vi "Project Step Operation.vi"(8 "error in (no error)":errorcluster, 9 "Drop Event Data":T1, 11 "Editor.lvclass in":refnum<data-value>) -> (0 "error out":errorcluster, 3 "Editor.lvclass out":refnum<data-value>)   [LabVIEW 2015, in "Editor.lvclass"]
uses:
  Editor.lvclass
  CallVIStep.lvclass
  CallEXEStep.lvclass
  UIStep.lvclass
  Project.lvclass
  Step.lvclass
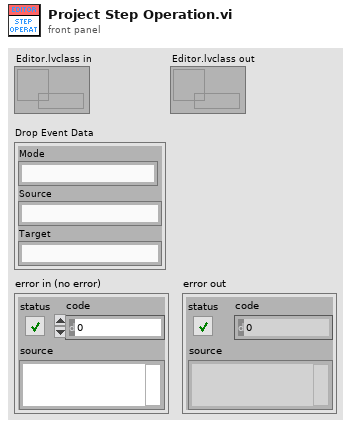
[diagram p1: front panel]
types:
  T1 = cluster{"Mode":string, "Source":string, "Target":string}
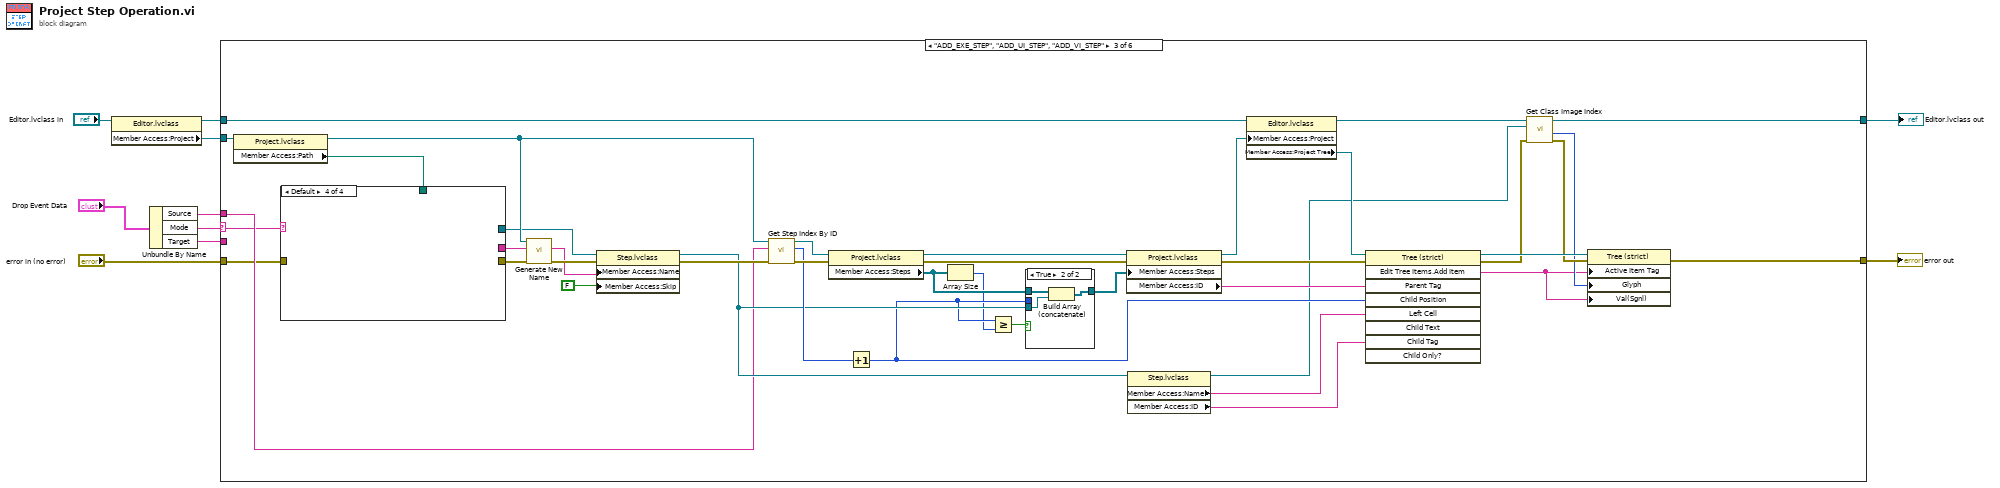
[diagram p0: block diagram]
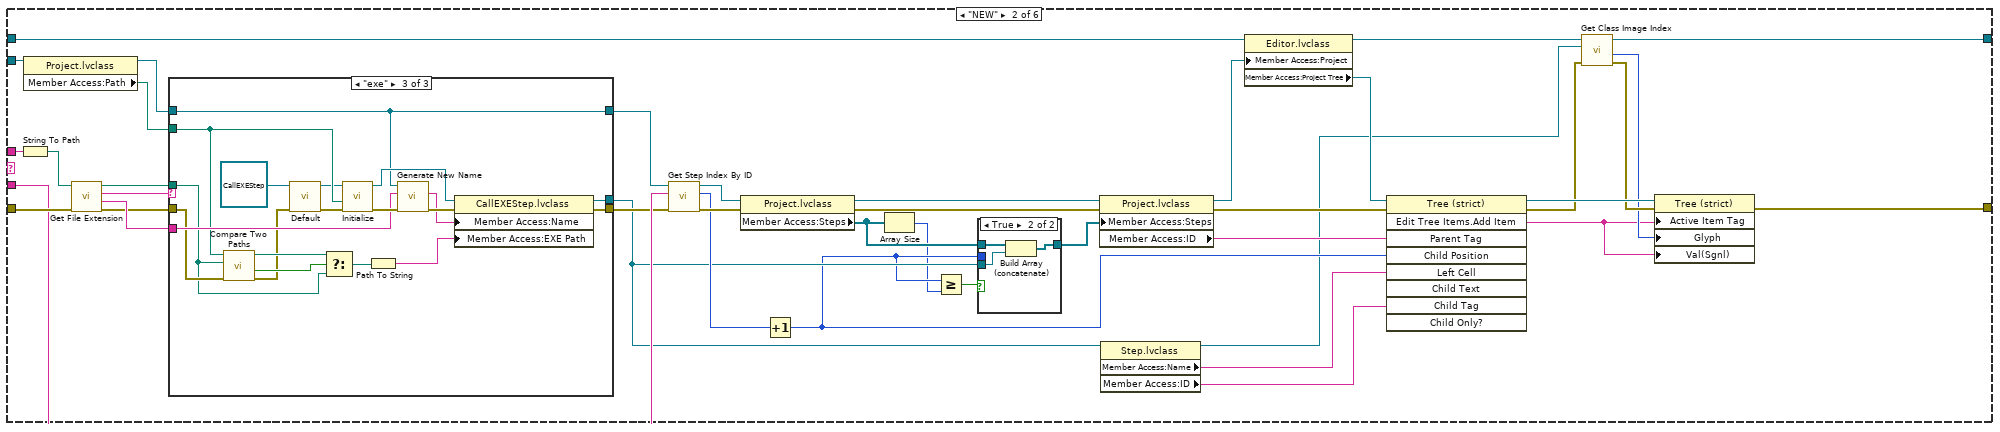
[diagram p3: hidden frame]
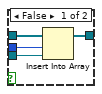
[diagram p4: hidden frame]
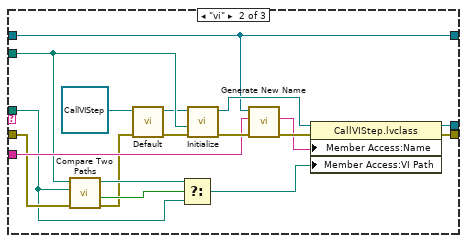
[diagram p6: hidden frame]
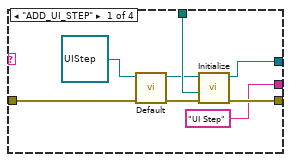
[diagram p7: hidden frame]
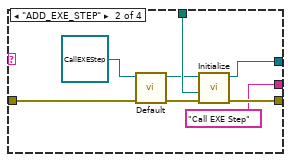
[diagram p8: hidden frame]
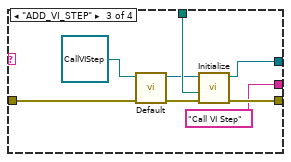
[diagram p9: hidden frame]
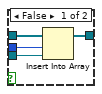
[diagram p10: hidden frame]
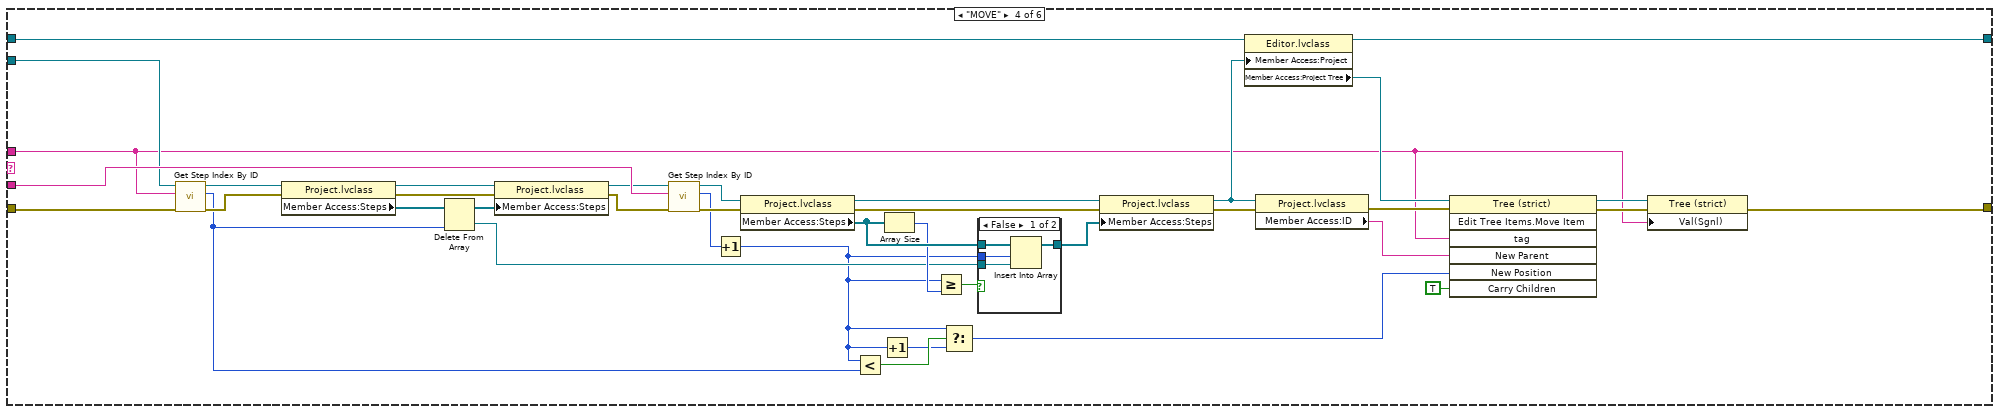
[diagram p11: hidden frame]
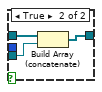
[diagram p12: hidden frame]
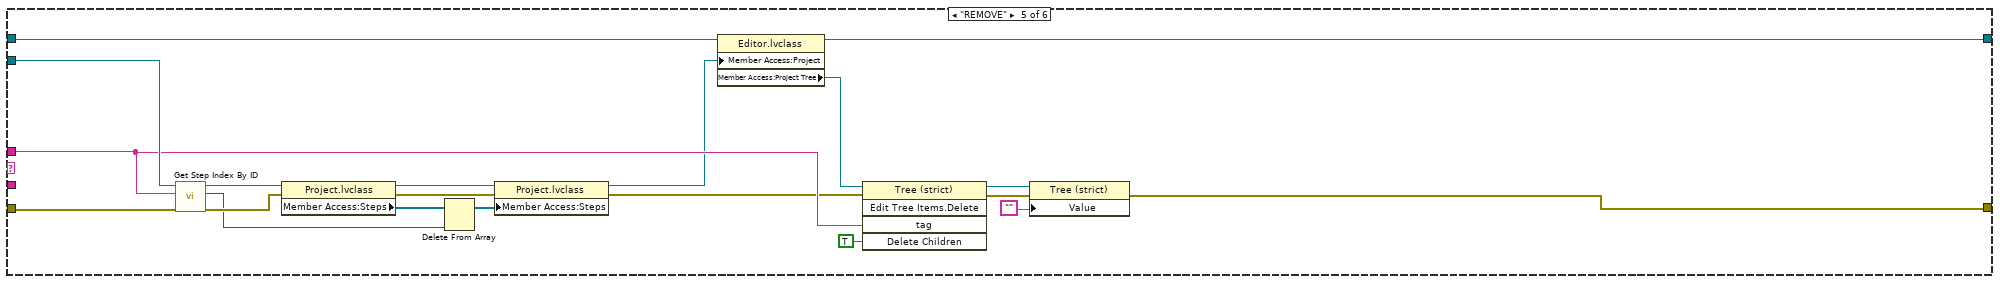
[diagram p13: hidden frame]
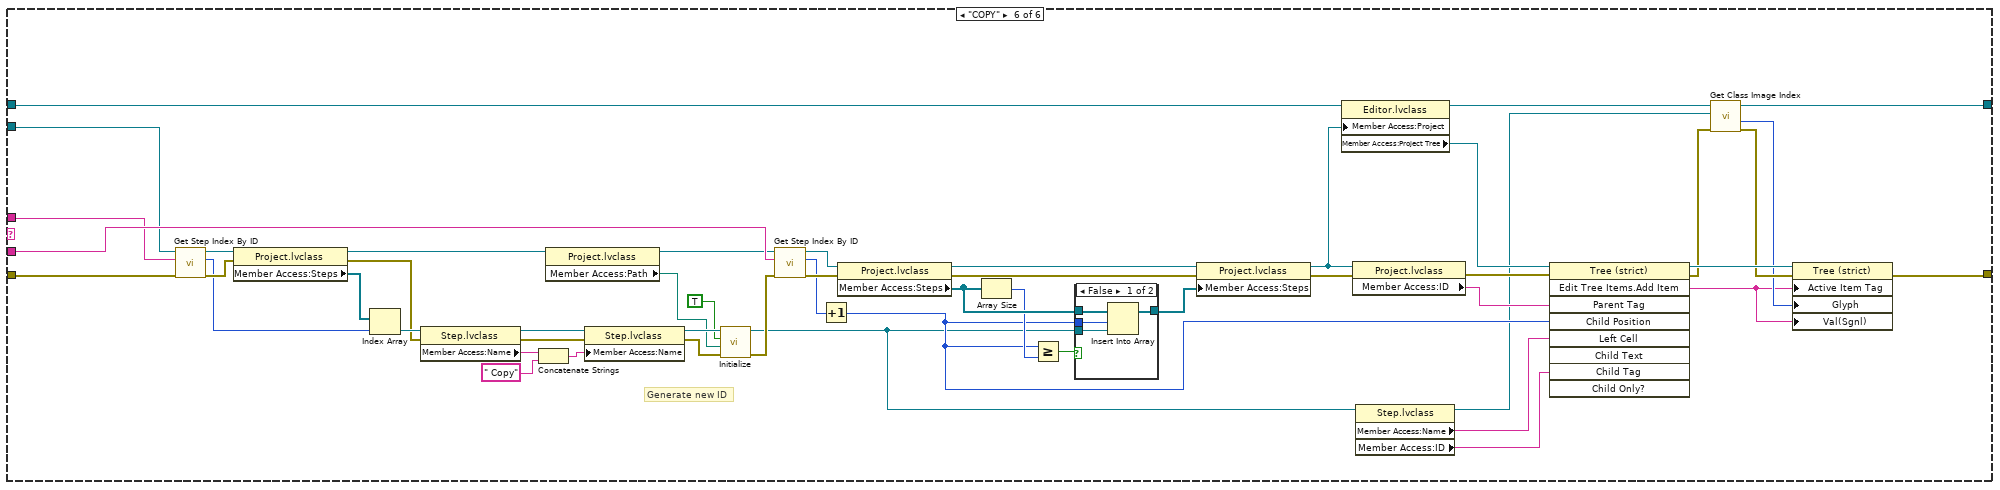
[diagram p14: hidden frame]
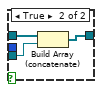
[diagram p15: hidden frame]
diagram:
  n1 = property class="Editor.lvclass"(reference="Editor.lvclass in") -> (reference out=w3:refnum<data-value>, "Member Access:Project"=w4:refnum<class "Project.lvclass">)  [unwired: 1 in, 1 out]
  n2 = Unbundle By Name("Drop Event Data") -> ("Source"=w8:string, "Mode"=w9:string, "Target"=w6:string)
  n3 = case shown="\"ADD_EXE_STEP\", \"ADD_UI_STEP\", \"ADD_VI_STEP\"" w9 {
    selector: w9 -> [_ _ w99 _ _ _]
    tunnel: w8 -> [_ w47 w102 w170 w219 w262]
    tunnel: w4 -> [_ w15 w109 w195 w232 w272]
    tunnel: "error in (no error)" -> [w11 w46 w100 w191 w228 w268]
    tunnel: w6 -> [_ w37 _ w200 _ w277]
    tunnel: w3 -> [w12 w45 w138 w207 w234 w284]
    tunnel: [w12 w17 w111 w184 w224 w242] -> w2
    tunnel: [w11 w16 w110 w171 w220 w263] -> w1
    frame Default {
    }
    frame "NEW" {
      n4 = String To Path(string=w47) -> (path=w48:path)
      n5 = property class="Project.lvclass"(reference=w15) -> (reference out=w14:refnum<class "Project.lvclass">, "Member Access:Path"=w13:path)  [unwired: 1 in, 1 out]
      n6 = call <vilib>:"Get File Extension.vi"("error in (no error)"=w46, "file"=w48) -> ("error out"=w50:errorcluster, "filename without extension"=w52:string, "lowercase file extension"=w49:string, "dup file"=w51:path)  [unwired: 5 in, 1 out]
      n7 = case shown="\"exe\"" w49 {
        tunnel: w50 -> [w61 w72 w91]
        tunnel: w51 -> [_ w67 w86]
        tunnel: [w61 w73 w92] -> w36
        tunnel: w14 -> [w60 w71 w90]
        tunnel: [w60 w71 w90] -> w38
        tunnel: w52 -> [_ w75 w94]
        tunnel: [_ w74 w93] -> w31
        tunnel: w13 -> [_ w70 w89]
        frame Default {
        }
        frame "vi" {
          n8 = call <vilib>:"Compare Two Paths.vi"("error in (no error)"=w72, "Path 2"=w67, "Path 1"=w70) -> ("error out"=w63:errorcluster, "Path 2 Relative to Path 1?"=w69:bool, "Relative Path from 1 to 2"=w68:path)  [unwired: 5 in, 1 out]
          n9 = call-dynamic "Default.vi"("error in (no error)"=w63, "CallVIStep in"=refnum<class "CallVIStep.lvclass"> refnum ("CallVIStep.lvclass")) -> ("error out"=w62:errorcluster, "CallVIStep out"=w64:refnum<class "CallVIStep.lvclass">)  [unwired: 8 in]
          n10 = Select(t=w68, s=w69, f=w67) -> (s? t:f=w66:path)
          n11 = call-dynamic "Initialize.vi"("error in (no error)"=w62, "Project Path"=w70, "Step in"=w64) -> ("error out"=w78:errorcluster, "Step out"=w79:refnum<class "CallVIStep.lvclass">)  [unwired: 7 in]
          n12 = call "Generate New Name.vi"("error in (no error)"=w78, "Default Name"=w75, "Project in"=w71) -> ("error out"=w77:errorcluster, "Name"=w76:string)  [unwired: 6 in, 1 out]
          n13 = property class="CallVIStep.lvclass"(reference=w79, error in=w77, "Member Access:Name"=w76, "Member Access:VI Path"=w66) -> (reference out=w74:refnum<class "CallVIStep.lvclass">, error out=w73:errorcluster)
        }
        frame "exe" {
          n14 = call <vilib>:"Compare Two Paths.vi"("error in (no error)"=w91, "Path 2"=w86, "Path 1"=w89) -> ("error out"=w81:errorcluster, "Path 2 Relative to Path 1?"=w87:bool, "Relative Path from 1 to 2"=w88:path)  [unwired: 5 in, 1 out]
          n15 = call-dynamic "Default.vi"("error in (no error)"=w81, "CallEXEStep in"=refnum<class "CallEXEStep.lvclass"> refnum ("CallEXEStep.lvclass")) -> ("error out"=w80:errorcluster, "CallEXEStep out"=w82:refnum<class "CallEXEStep.lvclass">)  [unwired: 8 in]
          n16 = Select(t=w88, s=w87, f=w86) -> (s? t:f=w85:path)
          n17 = call-dynamic "Initialize.vi"("error in (no error)"=w80, "Project Path"=w89, "Step in"=w82) -> ("error out"=w97:errorcluster, "Step out"=w98:refnum<class "CallEXEStep.lvclass">)  [unwired: 7 in]
          n18 = Path To String(path=w85) -> (string=w84:string)
          n19 = call "Generate New Name.vi"("error in (no error)"=w97, "Default Name"=w94, "Project in"=w90) -> ("error out"=w96:errorcluster, "Name"=w95:string)  [unwired: 6 in, 1 out]
          n20 = property class="CallEXEStep.lvclass"(reference=w98, error in=w96, "Member Access:Name"=w95, "Member Access:EXE Path"=w84) -> (reference out=w93:refnum<class "CallEXEStep.lvclass">, error out=w92:errorcluster)
        }
      }
      n21 = call "Get Step Index By ID.vi"("error in (no error)"=w36, "ID"=w37, "Project in"=w38) -> ("error out"=w41:errorcluster, "Index"=w40:i32, "Project out"=w42:refnum<class "Project.lvclass">)  [unwired: 6 in]
      n22 = property class="Project.lvclass"(reference=w42, error in=w41) -> (reference out=w44:refnum<class "Project.lvclass">, error out=w43:errorcluster, "Member Access:Steps"=w23:refnum<class "Step.lvclass">[])
      n23 = Increment(x=w40) -> (x+1=w21:i32)
      n24 = Array Size(array=w23) -> (size(s)=w20:i32)
      n25 = Greater Or Equal?(x=w21, y=w20) -> (x >= y?=w22:bool)
      n26 = case shown="True" w22 {
        tunnel: [w56 w57] -> w39
        tunnel: w31 -> [w55 w58]
        tunnel: w21 -> [w54 _]
        tunnel: w23 -> [w53 w59]
        frame False {
          n27 = Insert Into Array(array=w53, index=w54, new element=w55) -> (w56:refnum<class "Step.lvclass">[])
        }
        frame True {
          n28 = Build Array (concatenate)(w59, w58) -> (w57:refnum<class "Step.lvclass">[])
        }
      }
      n29 = property class="Project.lvclass"(reference=w44, error in=w43, "Member Access:Steps"=w39) -> (reference out=w35:refnum<class "Project.lvclass">, error out=w33:errorcluster, "Member Access:ID"=w32:string)
      n30 = property class="Step.lvclass"(reference=w31) -> (reference out=w18:refnum<class "Step.lvclass">, "Member Access:Name"=w30:string, "Member Access:ID"=w29:string)  [unwired: 1 in, 1 out]
      n31 = property class="Editor.lvclass"(reference=w45, "Member Access:Project"=w35) -> (reference out=w27:refnum<data-value>, "Member Access:Project Tree"=w34:refnum<vi>)  [unwired: 1 in, 1 out]
      n32 = invoke class="Tree (strict)" method="Edit Tree Items.Add Item"(reference=w34, error in=w33, "Parent Tag"=w32, "Child Position"=w21, "Left Cell"=w30, "Child Tag"=w29) -> (reference out=w28:refnum<vi>, error out=w26:errorcluster, "Edit Tree Items:Add Item"=w19:string)  [unwired: 3 in, 6 out]
      n33 = call "Get Class Image Index.vi"("error in (no error)"=w26, "SerializableObject in"=w18, "Editor.lvclass in"=w27) -> ("error out"=w25:errorcluster, "Index"=w24:i32, "Editor.lvclass out"=w17:refnum<data-value>)  [unwired: 5 in, 1 out]
      n34 = property class="Tree (strict)"(reference=w28, error in=w25, "Active Item Tag"=w19, "Glyph"=w24, "Val(Sgnl)"=w19) -> (error out=w16:errorcluster)  [unwired: 1 out]
    }
    frame "ADD_EXE_STEP", "ADD_UI_STEP", "ADD_VI_STEP" {
      n35 = property class="Project.lvclass"(reference=w109) -> (reference out=w131:refnum<class "Project.lvclass">, "Member Access:Path"=w108:path)  [unwired: 1 in, 1 out]
      n36 = case shown="Default" w99 {
        tunnel: w108 -> [w146 w154 w162 _]
        tunnel: [w145 w153 w161 _] -> w107
        tunnel: [w144 w152 w160 _] -> w105
        tunnel: ["UI Step" "Call EXE Step" "Call VI Step" _] -> w101
        tunnel: w100 -> [w140 w148 w156 _]
        frame "ADD_UI_STEP" {
          n37 = call-dynamic "Default.vi"("error in (no error)"=w140, "UIStep in"=refnum<class "UIStep.lvclass"> refnum ("UIStep.lvclass")) -> ("error out"=w139:errorcluster, "UIStep out"=w141:refnum<class "UIStep.lvclass">)  [unwired: 8 in]
          n38 = call-dynamic "Initialize.vi"("error in (no error)"=w139, "Project Path"=w146, "Step in"=w141) -> ("error out"=w144:errorcluster, "Step out"=w145:refnum<class "UIStep.lvclass">)  [unwired: 7 in]
        }
        frame "ADD_EXE_STEP" {
          n39 = call-dynamic "Default.vi"("error in (no error)"=w148, "CallEXEStep in"=refnum<class "CallEXEStep.lvclass"> refnum ("CallEXEStep.lvclass")) -> ("error out"=w147:errorcluster, "CallEXEStep out"=w149:refnum<class "CallEXEStep.lvclass">)  [unwired: 8 in]
          n40 = call-dynamic "Initialize.vi"("error in (no error)"=w147, "Project Path"=w154, "Step in"=w149) -> ("error out"=w152:errorcluster, "Step out"=w153:refnum<class "CallEXEStep.lvclass">)  [unwired: 7 in]
        }
        frame "ADD_VI_STEP" {
          n41 = call-dynamic "Default.vi"("error in (no error)"=w156, "CallVIStep in"=refnum<class "CallVIStep.lvclass"> refnum ("CallVIStep.lvclass")) -> ("error out"=w155:errorcluster, "CallVIStep out"=w157:refnum<class "CallVIStep.lvclass">)  [unwired: 8 in]
          n42 = call-dynamic "Initialize.vi"("error in (no error)"=w155, "Project Path"=w162, "Step in"=w157) -> ("error out"=w160:errorcluster, "Step out"=w161:refnum<class "CallVIStep.lvclass">)  [unwired: 7 in]
        }
        frame Default {
        }
      }
      n43 = call "Generate New Name.vi"("error in (no error)"=w105, "Default Name"=w101, "Project in"=w131) -> ("error out"=w104:errorcluster, "Name"=w103:string)  [unwired: 6 in, 1 out]
      n44 = property class="Step.lvclass"(reference=w107, error in=w104, "Member Access:Name"=w103, "Member Access:Skip"=FALSE ("Skip")) -> (reference out=w125:refnum<class "Step.lvclass">, error out=w130:errorcluster)
      n45 = call "Get Step Index By ID.vi"("error in (no error)"=w130, "ID"=w102, "Project in"=w131) -> ("error out"=w134:errorcluster, "Index"=w133:i32, "Project out"=w135:refnum<class "Project.lvclass">)  [unwired: 6 in]
      n46 = property class="Project.lvclass"(reference=w135, error in=w134) -> (reference out=w137:refnum<class "Project.lvclass">, error out=w136:errorcluster, "Member Access:Steps"=w117:refnum<class "Step.lvclass">[])
      n47 = Increment(x=w133) -> (x+1=w115:i32)
      n48 = Array Size(array=w117) -> (size(s)=w114:i32)
      n49 = Greater Or Equal?(x=w115, y=w114) -> (x >= y?=w116:bool)
      n50 = case shown="True" w116 {
        tunnel: [w166 w167] -> w132
        tunnel: w125 -> [w165 w168]
        tunnel: w115 -> [w164 _]
        tunnel: w117 -> [w163 w169]
        frame False {
          n51 = Insert Into Array(array=w163, index=w164, new element=w165) -> (w166:refnum<class "Step.lvclass">[])
        }
        frame True {
          n52 = Build Array (concatenate)(w169, w168) -> (w167:refnum<class "Step.lvclass">[])
        }
      }
      n53 = property class="Project.lvclass"(reference=w137, error in=w136, "Member Access:Steps"=w132) -> (reference out=w129:refnum<class "Project.lvclass">, error out=w127:errorcluster, "Member Access:ID"=w126:string)
      n54 = property class="Step.lvclass"(reference=w125) -> (reference out=w112:refnum<class "Step.lvclass">, "Member Access:Name"=w124:string, "Member Access:ID"=w123:string)  [unwired: 1 in, 1 out]
      n55 = property class="Editor.lvclass"(reference=w138, "Member Access:Project"=w129) -> (reference out=w121:refnum<data-value>, "Member Access:Project Tree"=w128:refnum<vi>)  [unwired: 1 in, 1 out]
      n56 = invoke class="Tree (strict)" method="Edit Tree Items.Add Item"(reference=w128, error in=w127, "Parent Tag"=w126, "Child Position"=w115, "Left Cell"=w124, "Child Tag"=w123) -> (reference out=w122:refnum<vi>, error out=w120:errorcluster, "Edit Tree Items:Add Item"=w113:string)  [unwired: 3 in, 6 out]
      n57 = call "Get Class Image Index.vi"("error in (no error)"=w120, "SerializableObject in"=w112, "Editor.lvclass in"=w121) -> ("error out"=w119:errorcluster, "Index"=w118:i32, "Editor.lvclass out"=w111:refnum<data-value>)  [unwired: 5 in, 1 out]
      n58 = property class="Tree (strict)"(reference=w122, error in=w119, "Active Item Tag"=w113, "Glyph"=w118, "Val(Sgnl)"=w113) -> (error out=w110:errorcluster)  [unwired: 1 out]
    }
    frame "MOVE" {
      n59 = call "Get Step Index By ID.vi"("error in (no error)"=w191, "ID"=w170, "Project in"=w195) -> ("error out"=w193:errorcluster, "Index"=w178:i32, "Project out"=w194:refnum<class "Project.lvclass">)  [unwired: 6 in]
      n60 = property class="Project.lvclass"(reference=w194, error in=w193) -> (reference out=w190:refnum<class "Project.lvclass">, error out=w188:errorcluster, "Member Access:Steps"=w192:refnum<class "Step.lvclass">[])
      n61 = Delete From Array(array=w192, index=w178) -> (deleted portion=w185:refnum<class "Step.lvclass">, array with subset deleted=w189:refnum<class "Step.lvclass">[])  [unwired: 1 in]
      n62 = property class="Project.lvclass"(reference=w190, error in=w188, "Member Access:Steps"=w189) -> (reference out=w187:refnum<class "Project.lvclass">, error out=w186:errorcluster)
      n63 = call "Get Step Index By ID.vi"("error in (no error)"=w186, "ID"=w200, "Project in"=w187) -> ("error out"=w203:errorcluster, "Index"=w202:i32, "Project out"=w204:refnum<class "Project.lvclass">)  [unwired: 6 in]
      n64 = Increment(x=w202) -> (x+1=w176:i32)
      n65 = property class="Project.lvclass"(reference=w204, error in=w203) -> (reference out=w206:refnum<class "Project.lvclass">, error out=w205:errorcluster, "Member Access:Steps"=w198:refnum<class "Step.lvclass">[])
      n66 = Less?(x=w176, y=w178) -> (x < y?=w177:bool)
      n67 = Increment(x=w176) -> (x+1=w175:i32)
      n68 = Array Size(array=w198) -> (size(s)=w196:i32)
      n69 = Greater Or Equal?(x=w176, y=w196) -> (x >= y?=w197:bool)
      n70 = Select(t=w176, s=w177, f=w175) -> (s? t:f=w174:i32)
      n71 = case shown="False" w197 {
        tunnel: [w211 w212] -> w201
        tunnel: w185 -> [w210 w213]
        tunnel: w176 -> [w209 _]
        tunnel: w198 -> [w208 w214]
        frame False {
          n72 = Insert Into Array(array=w208, index=w209, new element=w210) -> (w211:refnum<class "Step.lvclass">[])
        }
        frame True {
          n73 = Build Array (concatenate)(w214, w213) -> (w212:refnum<class "Step.lvclass">[])
        }
      }
      n74 = property class="Project.lvclass"(reference=w206, error in=w205, "Member Access:Steps"=w201) -> (reference out=w182:refnum<class "Project.lvclass">, error out=w181:errorcluster)
      n75 = property class="Editor.lvclass"(reference=w207, "Member Access:Project"=w182) -> (reference out=w184:refnum<data-value>, "Member Access:Project Tree"=w199:refnum<vi>)  [unwired: 1 in, 1 out]
      n76 = property class="Project.lvclass"(reference=w182, error in=w181) -> (error out=w180:errorcluster, "Member Access:ID"=w179:string)  [unwired: 1 out]
      n77 = invoke class="Tree (strict)" method="Edit Tree Items.Move Item"(reference=w199, error in=w180, "tag"=w170, "New Parent"=w179, "New Position"=w174, "Carry Children"=TRUE ("Carry Children?")) -> (reference out=w173:refnum<vi>, error out=w172:errorcluster)  [unwired: 1 in, 5 out]
      n78 = property class="Tree (strict)"(reference=w173, error in=w172, "Val(Sgnl)"=w170) -> (error out=w171:errorcluster)  [unwired: 1 out]
    }
    frame "REMOVE" {
      n79 = call "Get Step Index By ID.vi"("error in (no error)"=w228, "ID"=w219, "Project in"=w232) -> ("error out"=w230:errorcluster, "Index"=w223:i32, "Project out"=w231:refnum<class "Project.lvclass">)  [unwired: 6 in]
      n80 = property class="Project.lvclass"(reference=w231, error in=w230) -> (reference out=w227:refnum<class "Project.lvclass">, error out=w225:errorcluster, "Member Access:Steps"=w229:refnum<class "Step.lvclass">[])
      n81 = Delete From Array(array=w229, index=w223) -> (array with subset deleted=w226:refnum<class "Step.lvclass">[])  [unwired: 1 in, 1 out]
      n82 = property class="Project.lvclass"(reference=w227, error in=w225, "Member Access:Steps"=w226) -> (reference out=w218:refnum<class "Project.lvclass">, error out=w215:errorcluster)
      n83 = property class="Editor.lvclass"(reference=w234, "Member Access:Project"=w218) -> (reference out=w224:refnum<data-value>, "Member Access:Project Tree"=w233:refnum<vi>)  [unwired: 1 in, 1 out]
      n84 = invoke class="Tree (strict)" method="Edit Tree Items.Delete"(reference=w233, error in=w215, "tag"=w219, "Delete Children"=TRUE ("Delete Children?")) -> (reference out=w222:refnum<vi>, error out=w221:errorcluster)  [unwired: 1 in, 3 out]
      n85 = property class="Tree (strict)"(reference=w222, error in=w221, "Value"="") -> (error out=w220:errorcluster)  [unwired: 1 out]
    }
    frame "COPY" {
      # "Generate new ID"
      n86 = call "Get Step Index By ID.vi"("error in (no error)"=w268, "ID"=w262, "Project in"=w272) -> ("error out"=w270:errorcluster, "Index"=w261:i32, "Project out"=w271:refnum<class "Project.lvclass">)  [unwired: 6 in]
      n87 = property class="Project.lvclass"(reference=w271, error in=w270) -> (reference out=w237:refnum<class "Project.lvclass">, error out=w255:errorcluster, "Member Access:Steps"=w269:refnum<class "Step.lvclass">[])
      n88 = Index Array(array=w269, index=w261) -> (element=w260:refnum<class "Step.lvclass">)
      n89 = property class="Step.lvclass"(reference=w260, error in=w255) -> (reference out=w259:refnum<class "Step.lvclass">, error out=w252:errorcluster, "Member Access:Name"=w257:string)
      n90 = Concatenate Strings(w257, " Copy") -> (w258:string)
      n91 = property class="Project.lvclass"(reference=w237) -> (reference out=w236:refnum<class "Project.lvclass">, "Member Access:Path"=w235:path)  [unwired: 1 in, 1 out]
      n92 = property class="Step.lvclass"(reference=w259, error in=w252, "Member Access:Name"=w258) -> (reference out=w254:refnum<class "Step.lvclass">, error out=w253:errorcluster)
      n93 = call-dynamic "Initialize.vi"("error in (no error)"=w253, "Project Path"=w235, "New ID"=TRUE, "Step in"=w254) -> ("error out"=w251:errorcluster, "Step out"=w248:refnum<class "Step.lvclass">)  [unwired: 6 in]
      n94 = call "Get Step Index By ID.vi"("error in (no error)"=w251, "ID"=w277, "Project in"=w236) -> ("error out"=w280:errorcluster, "Index"=w279:i32, "Project out"=w281:refnum<class "Project.lvclass">)  [unwired: 6 in]
      n95 = Increment(x=w279) -> (x+1=w250:i32)
      n96 = property class="Project.lvclass"(reference=w281, error in=w280) -> (reference out=w283:refnum<class "Project.lvclass">, error out=w282:errorcluster, "Member Access:Steps"=w275:refnum<class "Step.lvclass">[])
      n97 = Array Size(array=w275) -> (size(s)=w273:i32)
      n98 = Greater Or Equal?(x=w250, y=w273) -> (x >= y?=w274:bool)
      n99 = case shown="False" w274 {
        tunnel: [w288 w289] -> w278
        tunnel: w248 -> [w287 w290]
        tunnel: w250 -> [w286 _]
        tunnel: w275 -> [w285 w291]
        frame False {
          n100 = Insert Into Array(array=w285, index=w286, new element=w287) -> (w288:refnum<class "Step.lvclass">[])
        }
        frame True {
          n101 = Build Array (concatenate)(w291, w290) -> (w289:refnum<class "Step.lvclass">[])
        }
      }
      n102 = property class="Project.lvclass"(reference=w283, error in=w282, "Member Access:Steps"=w278) -> (reference out=w267:refnum<class "Project.lvclass">, error out=w266:errorcluster)
      n103 = property class="Editor.lvclass"(reference=w284, "Member Access:Project"=w267) -> (reference out=w243:refnum<data-value>, "Member Access:Project Tree"=w276:refnum<vi>)  [unwired: 1 in, 1 out]
      n104 = property class="Project.lvclass"(reference=w267, error in=w266) -> (error out=w265:errorcluster, "Member Access:ID"=w249:string)  [unwired: 1 out]
      n105 = property class="Step.lvclass"(reference=w248) -> (reference out=w245:refnum<class "Step.lvclass">, "Member Access:Name"=w247:string, "Member Access:ID"=w246:string)  [unwired: 1 in, 1 out]
      n106 = invoke class="Tree (strict)" method="Edit Tree Items.Add Item"(reference=w276, error in=w265, "Parent Tag"=w249, "Child Position"=w250, "Left Cell"=w247, "Child Tag"=w246) -> (reference out=w264:refnum<vi>, error out=w244:errorcluster, "Edit Tree Items:Add Item"=w239:string)  [unwired: 3 in, 6 out]
      n107 = call "Get Class Image Index.vi"("error in (no error)"=w244, "SerializableObject in"=w245, "Editor.lvclass in"=w243) -> ("error out"=w241:errorcluster, "Index"=w240:i32, "Editor.lvclass out"=w242:refnum<data-value>)  [unwired: 5 in, 1 out]
      n108 = property class="Tree (strict)"(reference=w264, error in=w241, "Active Item Tag"=w239, "Glyph"=w240, "Val(Sgnl)"=w239) -> (error out=w263:errorcluster)  [unwired: 1 out]
    }
  }
  "error out" <- w1
  "Editor.lvclass out" <- w2
